vi "Read-all-gui-params.vi"(8 "error in (no error)":errorcluster, 11 "Correct. params. ref. in":refnum<data-value>) -> (0 "error out":errorcluster, 2 "Correction params.":T1={"Background correction"=FALSE, "Hot-pixel correction"=FALSE, "Black image cam. 1"=path "C:/CameraVision/Black images/Black-CameraA-Full.bmp", "Black image cam. 2"=path "C:/CameraVision/Black images/Black-CameraB-Full.bmp", "Y-shift"=0, "X-shift"=0, "Correlation algorithm"=enum."Fixed shift", "Noise treshold"=25.0, "Smoothing algorithm"=enum."Noise tresholding", "2nd image correlation"=FALSE, "Image smoothing"=FALSE, "Background correction method"=enum."Hardware"} {"Noise treshold" min=0 max=255 step=1}, 3 "Correct. params. ref.":refnum<data-value>)   [LabVIEW 2013, in "CameraVision.lvlib" / "CV-Correction.lvclass"]
uses:
  CV-Correction.lvclass
  Correction-parameters-gui.ctl
  Smoothing.ctl
  Background-correction.ctl
  CV-Correction.lvclass/CV-Correction.ctl
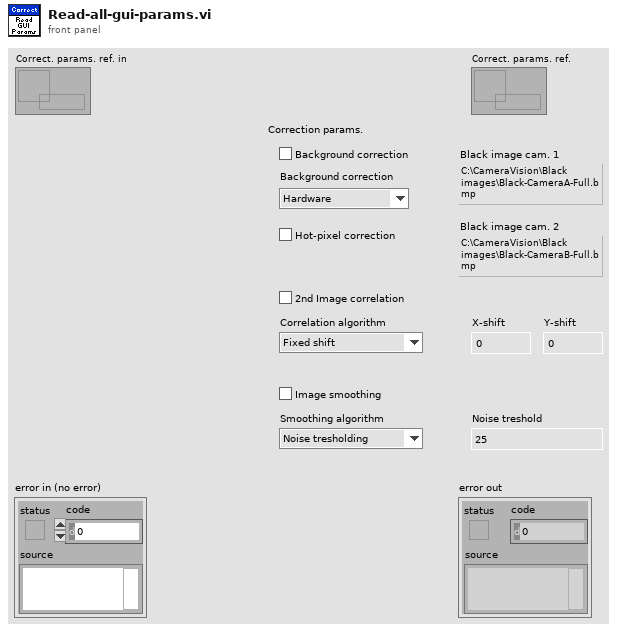
[diagram p1: front panel]
types:
  T1 = typedef "CameraVision.lvlib/CV-Correction.lvclass/Correction-parameters-gui.ctl" = cluster{"Background correction":bool, "Hot-pixel correction":bool, "Black image cam. 1":path, "Black image cam. 2":path, "Y-shift":i32, "X-shift":i32, "Correlation algorithm":enum16{"Fixed shift", "Cross-correlation", "Cross-correlation (5steps)", "Melt-pool center"}, "Noise treshold":sgl, "Smoothing algorithm":T2, "2nd image correlation":bool, "Image smoothing":bool, "Background correction method":T3}
  T2 = typedef "CameraVision.lvlib/CV-Correction.lvclass/Smoothing.ctl" = enum16{"Noise tresholding", "NT+Median filter", "NT+Gaussian filter"}
  T3 = typedef "CameraVision.lvlib/CV-Correction.lvclass/Background-correction.ctl" = enum16{"Hardware", "Software"}
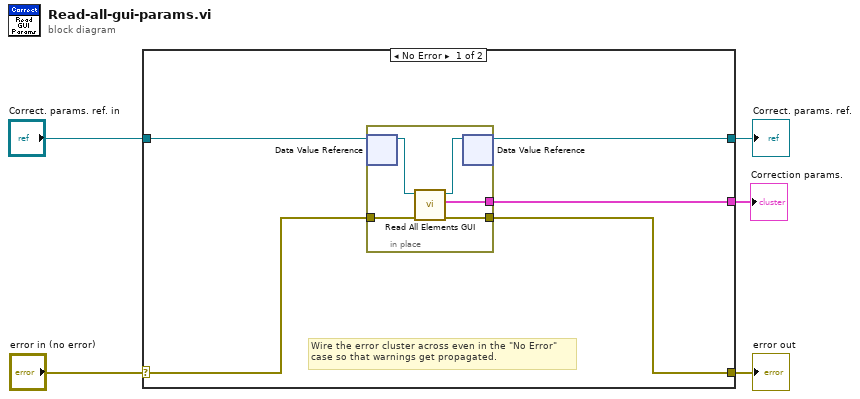
[diagram p0: block diagram]
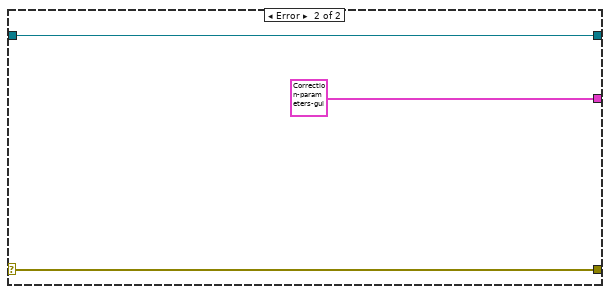
[diagram p2: hidden frame]
diagram:
  n1 = case shown="No Error" "error in (no error)" {
    selector: "error in (no error)" -> [w8 w18]
    tunnel: [w10 w18] -> w4
    tunnel: "Correct. params. ref. in" -> [w7 w16]
    tunnel: [w9 T1 {"Background correction"=FALSE, "Hot-pixel correction"=FALSE, "Black image cam. 1"=path "C:/CameraVision/Black images/Black-CameraA-Full.bmp", "Black image cam. 2"=path "C:/CameraVision/Black images/Black-CameraB-Full.bmp", "Y-shift"=0, "X-shift"=0, "Correlation algorithm"=enum."Fixed shift", "Noise treshold"=25.0, "Smoothing algorithm"=enum."Noise tresholding", "2nd image correlation"=FALSE, "Image smoothing"=FALSE, "Background correction method"=enum."Hardware"} ("Correction params.")] -> w2
    tunnel: [w6 w16] -> w1
    frame No Error {
      # "Wire the error cluster across even in the \"No Error\"\ncase so that warnings get propagated."
      n2 = in-place {
        in-place-border: [w15] -> w10
        in-place-border: [w14] -> w9
        in-place-border: w8 -> [w13]
        n3 = in-place-dvr #1(w7) -> (w12:refnum<class "CV-Correction.lvclass">)  [unwired: 1 out]
        n4 = call "Read All Elements GUI.vi"("error in (no error)"=w13, "Correct params in"=w12) -> ("error out"=w15:errorcluster, "Correction params."=w14:T1, "Correct params out"=w11:refnum<class "CV-Correction.lvclass">)  [unwired: 7 in]
        n5 = in-place-dvr #1(w11) -> (w6:refnum<data-value>)  [unwired: 1 out]
      }
    }
    frame Error {
    }
  }
  "error out" <- w4
  "Correct. params. ref." <- w1
  "Correction params." <- w2
